vi "filterWheelThorlabsOpen.vi"   [LabVIEW 2017]
uses:
  globalDevices.vi
  <vilib>/Instr/_visa.llb/VISA Configure Serial Port (Instr).vi
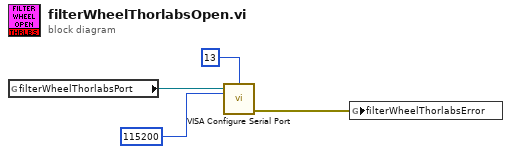
[diagram p0: block diagram]
diagram:
  n1 = global read "globalDevices.vi" "filterWheelThorlabsPort"() -> (w3:refnum<visa-resource-name>)
  n2 = call-poly "VISA Configure Serial Port"("VISA resource name"=w3, "termination char\n(0xA = '\\n' = LF)"=u8 13 ("termination char\n(0xA = '\\n' = LF)"), "baud rate (9600)"=u32 115200) -> ("error out"=w1:errorcluster)  [unwired: 11 in, 1 out]
  n3 = global write "globalDevices.vi" "filterWheelThorlabsError"(w1) -> ()
